vi "Launcher.vi"() -> ()   [LabVIEW 2014, in "HIJ Vision App IMAQdx Display.lvlib"]
uses:
  HIJ Vision App IMAQdx Display.lvlib
  <vilib>/userdefined/High Color/IMAQdx.ctl
  HIJ Vision App IMAQdx Display/HIJ Vision App IMAQdx Display.lvclass
  <vilib>/Utility/config.llb/Read Key (Path).vi
  <vilib>/Utility/config.llb/Read Key (String).vi
  HIJ Vision Camera App/HIJ Vision Camera App/Write Start Camera.vi
  HIJ Vision Camera App/HIJ Vision Camera App/Write my ConfigDir.vi
  HIJ Vision Camera App/HIJ Vision Camera App/Write my WorkDir.vi
  HIJ Vision Camera App/HIJ Vision Camera App/Write Start Acquisition.vi
  <vilib>/Utility/config.llb/Write Key (Path).vi
  <vilib>/Utility/config.llb/Write Key (String).vi
  <vilib>/ActorFramework/Actor/Actor.lvclass
  <vilib>/Utility/config.llb/NI_LVConfig.lvlib
panel:
  in  "UI Cnfg":path
  in  "CLine Parameter":string
  in  "RUN_STOP":bool=TRUE
  in  "Start WorkDir":path=path "C:/Users/user/Desktop/test/WorkDir"
  in  "Start ConfigDir":path=path "C:/Users/user/Desktop/test/ConfigDir"
  in  "Start Camera":T1="TestCam"
  out "error out":errorcluster
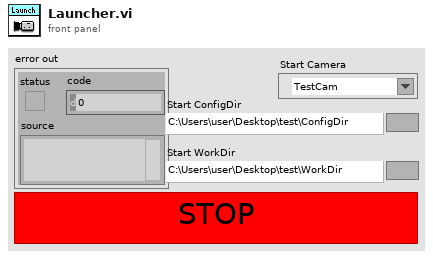
[diagram p1: front panel]
types:
  T1 = typedef "IMAQdx.ctl" = refnum<k21>
  T2 = typedef "NI_LVConfig.lvlib/Config Data RefNum.ctl" = refnum<k1>
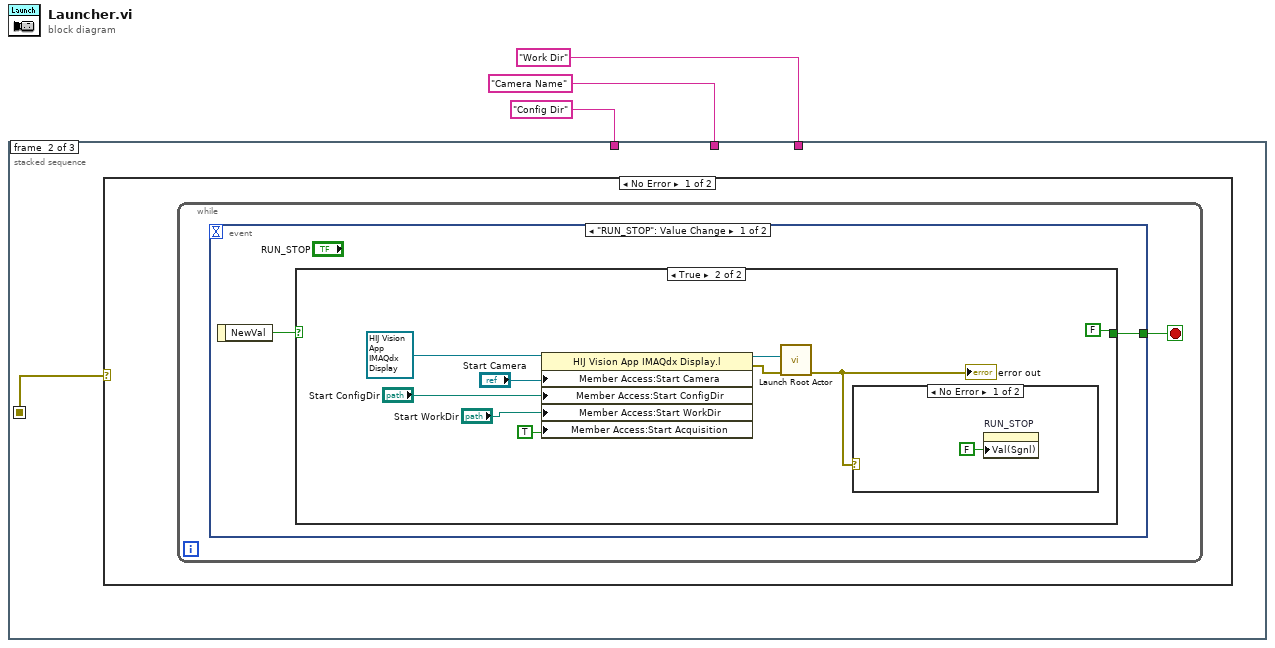
[diagram p0: block diagram]
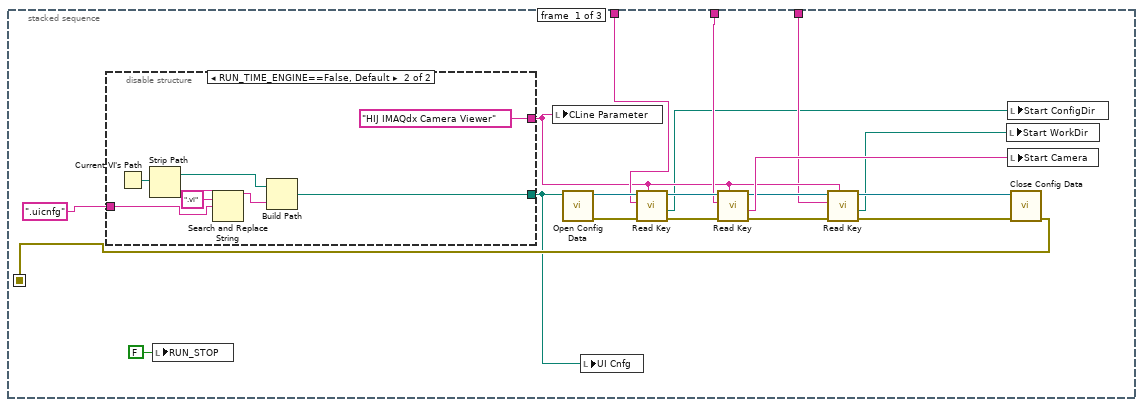
[diagram p2: hidden frame]
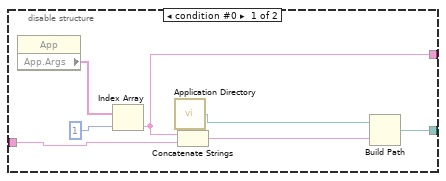
[diagram p3: hidden frame]
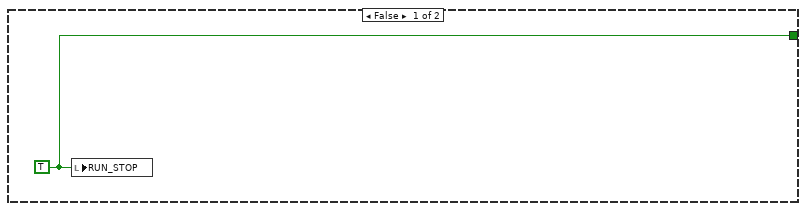
[diagram p4: hidden frame]
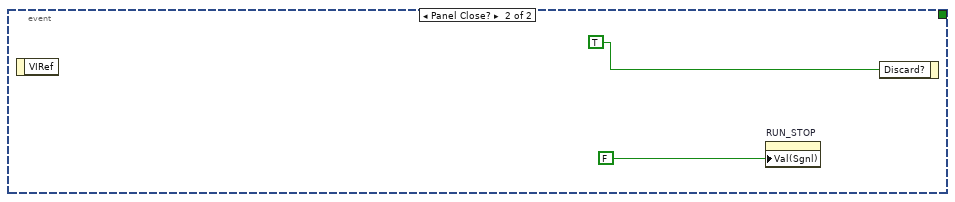
[diagram p6: hidden frame]
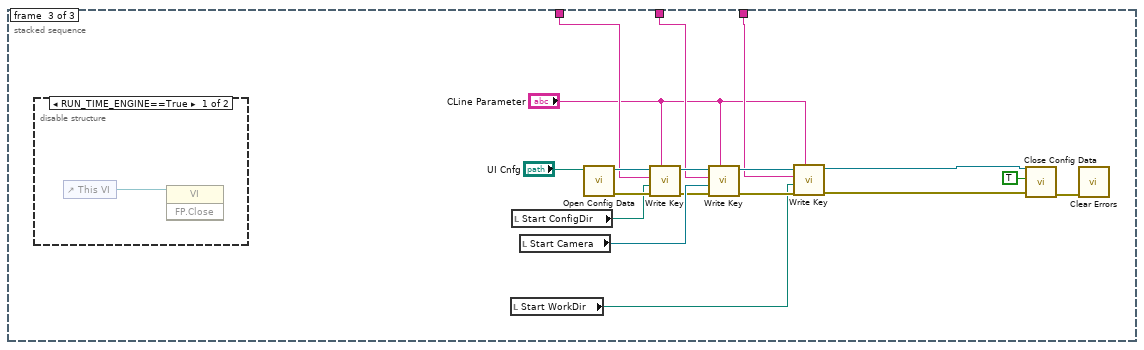
[diagram p8: hidden frame]
diagram:
  n1 = stacked-sequence {
    seq-local: [w15 _ _] -> [_ w38 _]
    tunnel: "Camera Name" ("key") -> [w17 _ w68]
    tunnel: "Config Dir" ("key") -> [w16 _ w69]
    tunnel: "Work Dir" ("key") -> [w6 _ w56]
    frame #0 {
      n2 = disable-structure shown="RUN_TIME_ENGINE==False, Default" {
        disable-tunnel: [w25 w31] -> w13
        disable-tunnel: ".uicnfg" ("string") -> [w24 w34]
        disable-tunnel: [w23 "HIJ IMAQdx Camera Viewer"] -> w7
        frame condition #0 {
          n3 = property class="App"() -> ("App.Args"=w29:string[])  [unwired: 2 in, 2 out]
          n4 = Index Array(array=w29, index=1) -> (element=w23:string)
          n5 = call <vilib>:"Application Directory.vi"() -> ("Application Directory"=w27:path)
          n6 = Concatenate Strings(w23, w24) -> (w26:string)
          n7 = Build Path(base path=w27, name or relative path=w26) -> (appended path=w25:path)
        }
        frame condition #1 (active) {
          n8 = Current VI's Path() -> (path=w37:path)
          n9 = Strip Path(path=w37) -> (stripped path=w32:path, name=w36:string)
          n10 = Search and Replace String(input string=w36, search string=".vi", replace string=w34) -> (result string=w33:string)  [unwired: 5 in, 3 out]
          n11 = Build Path(base path=w32, name or relative path=w33) -> (appended path=w31:path)
        }
      }
      n12 = local write "RUN_STOP"(FALSE ("RUN_STOP")) -> ()
      n13 = local write "CLine Parameter"(w7) -> ()
      n14 = call <vilib>:"Open Config Data.vi"("configuration file path"=w13) -> ("error out"=w19:errorcluster, "refnum"=w18:T2)  [unwired: 8 in, 1 out]
      n15 = local write "UI Cnfg"(w13) -> ()
      n16 = call-poly <vilib>:"Read Key.vi"("section"=w7, "error in (no error)"=w19, "key"=w16, "refnum"=w18) -> ("error out"=w20:errorcluster, "value"=w4:path, "refnum out"=w21:T2)  [unwired: 4 in, 1 out]
      n17 = call-poly <vilib>:"Read Key.vi"("section"=w7, "error in (no error)"=w20, "key"=w17, "refnum"=w21) -> ("error out"=w11:errorcluster, "value"=w12:string, "refnum out"=w9:T2)  [unwired: 4 in, 1 out]
      n18 = call-poly <vilib>:"Read Key.vi"("section"=w7, "error in (no error)"=w11, "key"=w6, "refnum"=w9) -> ("error out"=w10:errorcluster, "value"=w5:path, "refnum out"=w8:T2)  [unwired: 4 in, 1 out]
      n19 = local write "Start WorkDir"(w5) -> ()
      n20 = local write "Start ConfigDir"(w4) -> ()
      n21 = local write "Start Camera"(w12) -> ()
      n22 = call <vilib>:"Close Config Data.vi"("error in (no error)"=w10, "refnum"=w8) -> ("error out"=w15:errorcluster)  [unwired: 8 in, 1 out]
    }
    frame #1 {
      n23 = case shown="No Error" w38 {
        frame No Error {
          n24 = while {
            stop <- w39 stop-if-true
            n25 = event shown="[0] \"RUN_STOP\": Value Change" {
              selector: _ -> [_ _]
              dyn-events: _ -> [_ _]
              timeout: _ -> [_ _]
              tunnel: [w41 _] -> w39
              event "RUN_STOP": Value Change {
                n26 = event-data() -> ("NewVal"=w40:bool)  [unwired: 1 in]
                n27 = case shown="True" w40 {
                  tunnel: [w42 FALSE] -> w41
                  frame False {
                    w42 = TRUE ("RUN_STOP")
                    n28 = local write "RUN_STOP"(w42) -> ()
                  }
                  frame True {
                    n29 = property class="HIJ Vision App IMAQdx Display.l"(reference=refnum<class "HIJ Vision App IMAQdx Display.lvclass"> refnum ("Launch IMAQ Display.lvlib:Launch IMAQ Display.lvclass"), "Member Access:Start Camera"="Start Camera", "Member Access:Start ConfigDir"="Start ConfigDir", "Member Access:Start WorkDir"="Start WorkDir", "Member Access:Start Acquisition"=TRUE ("Start Acquisition")) -> (reference out=w45:refnum<class "HIJ Vision App IMAQdx Display.lvclass">, error out=w46:errorcluster)  [unwired: 1 in]
                    n30 = call <vilib>:"Launch Root Actor.vi"("error in (no error)"=w46, "Actor"=w45) -> ("error out"=w43:errorcluster)  [unwired: 8 in, 1 out]
                    "error out" <- w43
                    n31 = case shown="No Error" w43 {
                      frame No Error {
                        n32 = property on="RUN_STOP" class="Bool (strict)"("Val(Sgnl)"=FALSE ("Value (Signaling)")) -> ()  [unwired: 2 in, 2 out]
                      }
                      frame Error {
                      }
                    }
                  }
                }
              }
              event Panel Close? {
                n33 = event-data() -> ()  [unwired: 1 in, 1 out]
                n34 = property on="RUN_STOP" class="Bool (strict)"("Val(Sgnl)"=FALSE ("Value (Signaling)")) -> ()  [unwired: 2 in, 2 out]
                n35 = event-data("Discard?"=TRUE) -> ()  [unwired: 1 in, 1 out]
              }
            }
          }
        }
        frame Error {
        }
      }
    }
    frame #2 {
      n36 = disable-structure shown="RUN_TIME_ENGINE==True" {
        frame condition #0 {
          n37 = control-ref of="This VI"() -> (w73:refnum<vi>)
          n38 = invoke class="VI" method="FP.Close"(reference=w73) -> ()  [unwired: 2 in, 3 out]
        }
        frame condition #1 (active) {
        }
      }
      n39 = local read "Start WorkDir"() -> (w57:path)
      n40 = local read "Start ConfigDir"() -> (w62:path)
      n41 = local read "Start Camera"() -> (w67:T1)
      n42 = call <vilib>:"Open Config Data.vi"("configuration file path"="UI Cnfg") -> ("error out"=w66:errorcluster, "refnum"=w71:T2)  [unwired: 8 in, 1 out]
      n43 = call-poly <vilib>:"Write Key.vi"("section"="CLine Parameter", "error in (no error)"=w66, "value"=w62, "key"=w69, "refnum"=w71) -> ("error out"=w65:errorcluster, "refnum out"=w72:T2)  [unwired: 4 in, 1 out]
      n44 = call-poly <vilib>:"Write Key.vi"("section"="CLine Parameter", "error in (no error)"=w65, "value"=w67, "key"=w68, "refnum"=w72) -> ("error out"=w60:errorcluster, "refnum out"=w61:T2)  [unwired: 4 in, 1 out]
      n45 = call-poly <vilib>:"Write Key.vi"("section"="CLine Parameter", "error in (no error)"=w60, "value"=w57, "key"=w56, "refnum"=w61) -> ("error out"=w59:errorcluster, "refnum out"=w58:T2)  [unwired: 4 in, 1 out]
      n46 = call <vilib>:"Close Config Data.vi"("error in (no error)"=w59, "write file if changed (T)"=TRUE, "refnum"=w58) -> ("error out"=w64:errorcluster)  [unwired: 7 in, 1 out]
      n47 = call <vilib>:"Clear Errors.vi"("error in (no error)"=w64) -> ()  [unwired: 5 in, 2 out]
    }
  }
